vi "QUBE-Servo 2 ROTPEN LQR Design.vi"() -> ()   [LabVIEW 2016]
uses:
  <vilib>/addons/Control Design/_Model Construction/Model File IO.llb/Model File IO Subvi/cd_Read Model from File (SS).vi
  <vilib>/addons/Control Design/_Dynamic Analysis/Dynamic Analysis.llb/Dynamic Analysis subVI/cd_Poles (State-Space).vi
  <vilib>/addons/Control Design/_Utility/Model Viewer.llb/Model Viewer SubVI/cd_Draw State-Space Equation (SS).vi
  <vilib>/addons/Control Design/_State Feedback Control/State Feedback Control.llb/State Feedback Control SubVis/cd_Linear Quadratic Regulator.vi
  <vilib>/addons/Control Design/_Model Construction/NI_LinSys_Model File IO.lvlib
  <vilib>/addons/Control Design/_Utility/NI_CD_Model Viewer.lvlib
  <vilib>/addons/Control Design/_State Feedback Control/NI_CD_State Feedback Control.lvlib
  <vilib>/addons/Control Design/_Dynamic Analysis/NI_CD_Dynamic Analysis.lvlib
panel:
  out "Feedback Gain K":dbl[][](array[numeric])=[[-1.3003924395663553], [5.645628813133262], [-0.5689370850408126], [0.7658149722138641]] format="%.2f"
  in  "R":dbl[][](array[numeric])=[[1.0]] format="%.2f"
  in  "Q":dbl[][](array[numeric])=[[1.0, 0.0, 0.0, 0.0], [0.0, 1.0, 0.0, 0.0], [0.0, 0.0, 1.0, 0.0], [0.0, 0.0, 0.0, 1.0]] format="%.2f"
  out "Poles":cdb[](array[numeric]) format="%.3f"
  out "Open Loop State-Space Model":picture
  in  "File Path (dialog if empty)":path
  # "Rotary Motion Platform"
  # "QUBE-Servo 2 | LQR Design"
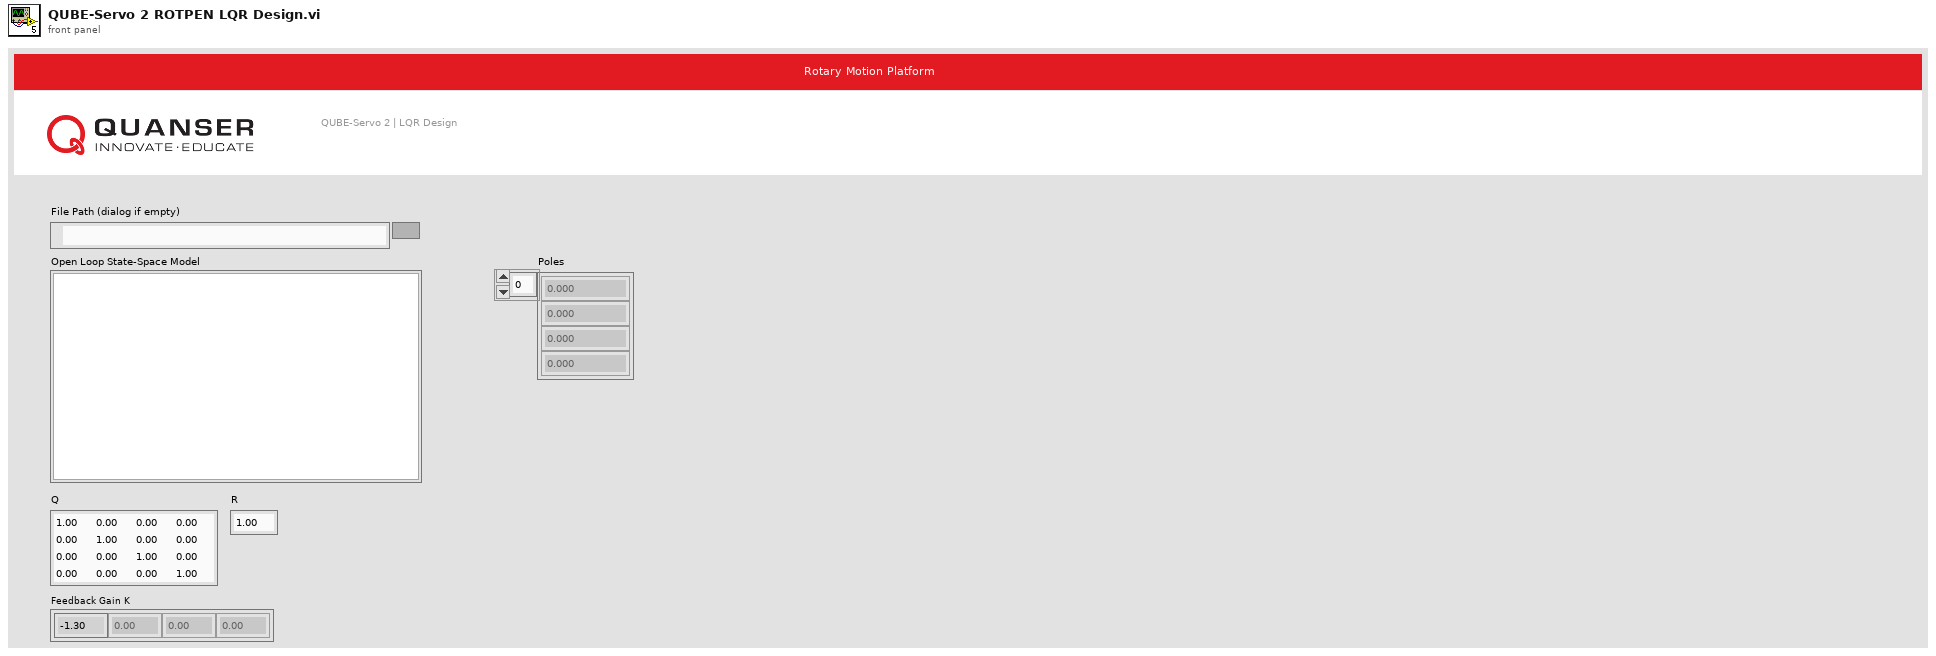
[diagram p1: front panel]
types:
  T1 = typedef "NI_LinSys_Model Typedefs.lvlib/CD State Space Model (MIMO).ctl" = cluster{"properties":T2, "A":dbl[][], "B":dbl[][], "C":dbl[][], "D":dbl[][], "StateNames":string[], "Transport Delay":dbl[][]}
  T2 = typedef "NI_LinSys_Model Typedefs.lvlib/CD General Elements.ctl" = cluster{"Model name":string, "Input names":string[], "Output names":string[], "Input Delays":dbl[], "Output Delays":dbl[], "Sampling Time":dbl, "Notes":string}
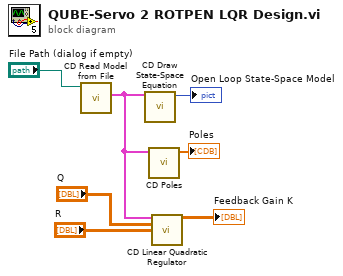
[diagram p0: block diagram]
diagram:
  n1 = call-poly <vilib>:"CD Read Model from File.vi"("File Path (dialog if empty)"="File Path (dialog if empty)") -> ("First State-Space Model in Record"=w4:T1)  [unwired: 6 in, 4 out]
  n2 = call-poly <vilib>:"CD Draw State-Space Equation.vi"("State-Space Model"=w4) -> ("Equation"=→"Open Loop State-Space Model":picture)  [unwired: 8 in, 2 out]
  n3 = call-poly <vilib>:"CD Poles.vi"("State-Space Model"=w4) -> ("Poles"=→"Poles":cdb[])  [unwired: 9 in, 1 out]
  n4 = call-poly <vilib>:"CD Linear Quadratic Regulator.vi"("State-Space Model"=w4, "Q"="Q", "R"="R") -> ("Optimal Gain (K)"=→"Feedback Gain K":dbl[][])  [unwired: 9 in, 3 out]
